vi "Log Data.vi"(8 "error in (no error)":errorcluster, 9 "DataQueues":refnum<queue>[](array[refnum]), 10 "UI":refnum<queue>, 11 "Config":T1={"Hardware Configuration"={"Camera Configuration"={"Setting"={"Expouse"=0.0, "Frames"=0.0, "Interval"=0.0, "ROI"={"x"=0.0, "y"=0.0, "width"=0.0, "height"=0.0}, "Binning"={"Binning X"=0.0, "Binning Y"=0.0}}, "Resource"={"CameraRef"=refnum, "LibraryRef"=refnum, "ImagesArray"=[]}}, "Stages Configuration"={"Resource"={"NanoStage Ref"=0, "MicroStage Ref"=0, "TirfLock Ref"=0}, "SettingValues"={"NanoState"={"Time"=0.0, "X"=0.0, "Y"=0.0, "Z"=0.0}, "MicroState"={"Time 2"=0.0, "Z"=0.0, "IsEPISet?"=FALSE}, "TirfLock"={"Time"=0.0, "X"=0.0, "Y"=0.0, "Sum"=0.0, "Calbrate"=0.0, "LockedTarget"=0.0, "Kp"=0.0, "Ki"=0.0, "Avg"=0.0}}}, "Lasers Configuration"={"SettingValues"={"405 Power"=0.0, "488 Power"=0.0, "532 Power"=0.0, "561 Power"=0.0, "647 Power"=0.0, "785 Power"=0.0}, "Resource"={"Library Ref"=refnum, "Lasers Ref"={"405 Ref"=refnum, "488 Ref"=refnum, "532 Ref"=refnum, "561 Ref"=refnum, "647 Ref"=refnum, "785 Ref"=refnum}}}}, "Logging Configuration"={"Log File Base Folder"=path "", "FileSurfix"="", "TiffFileFullPath"=path "", "TimeStampFile Ref"=refnum, "NoteFileRef"=refnum, "QuickNoteInfo"=""}, "HardWare Status"={"CameraAndStages"={"Camera"=FALSE, "NanoStage"=FALSE, "MicroStage"=FALSE, "TIRFLock"=FALSE}, "Lasers"={"IsConnected"={"405"=FALSE, "488"=FALSE, "532"=FALSE, "561"=FALSE, "647"=FALSE, "785"=FALSE}, "IsOpened"={"405"=FALSE, "488"=FALSE, "532"=FALSE, "561"=FALSE, "647"=FALSE, "785"=FALSE}}}, "CallBack Ref"={"LiveAcq callback Ref"=refnum, "AlbumAcq callback Ref"=refnum, "SequenceAcq callback Ref"=refnum, "Camera Status callback Ref"=refnum}, "Acqusition Control"={"Images Saving"={"StreamToDisk?"=FALSE, "SingleStack?"=FALSE, "Alert when finish?"=FALSE}, "Debug"={"Global Debug"=FALSE, "Global Debug Value"=0.0}}, "Runtime Parameters"={"Scale Bar"=TRUE, "ScaleBarSize"=10.0, "XYIncreatement+"=40.0, "ZIncreatement++"=5.0, "Autostretch"=FALSE, "ZIncreatement+"=0.2, "MicroStage+"=100.0, "XYIncreatement++"=80.0}} {"Runtime Parameters"."XYIncreatement++" format="%#_13g"; "Runtime Parameters"."MicroStage+" format="%#_13g"; "Runtime Parameters"."ZIncreatement+" format="%#_13g"; "Runtime Parameters"."ZIncreatement++" format="%#_13g"; "Runtime Parameters"."XYIncreatement+" format="%#_13g"; "Runtime Parameters"."ScaleBarSize" format="%#_13g"; "Hardware Configuration"."Lasers Configuration"."SettingValues"."785 Power" format="%.1f"; "Hardware Configuration"."Lasers Configuration"."SettingValues"."647 Power" format="%.1f"; "Hardware Configuration"."Lasers Configuration"."SettingValues"."561 Power" format="%.1f"}) -> (0 "error out":errorcluster)   [LabVIEW 2020, in "Logging.lvlib"]
doc: "This VI uses the TDMS Write function to write data to a TDMS file."
uses:
  Logging.lvlib
  Settings/System Running Settings.ctl
  HardwareAdapter/Support/Hardware Configuration.ctl
  HardwareAdapter/Support/Camera Configuration.ctl
  controls/ROI.ctl
  D:/Daguan/Development/RM21-MMicrosopeSource/HardwareAdapter/Camera/Dependencies/PVCamNET.dll
  HardwareAdapter/Camera/Dependencies/PVCamNET.dll
  <vilib>/vision/Image Controls.llb/IMAQ Image.ctl
  D:/Daguan/Development/RM21-MMicrosopeSource/HardwareAdapter/Lasers/Dependencies/Oxxius_Boxx.dll
  HardwareAdapter/Lasers/Dependencies/Oxxius_Boxx.dll
  Logging Configuration.ctl
  controls/DeviceStatusCtl.ctl
  controls/CallBack Refs.ctl
  Acquisition/Acquisition Control.ctl
  controls/Runtime Parameters.ctl
  support/Message Queue/Message Cluster.ctl
  controls/Image MatadataCtl.ctl
  Global.vi
  Settings/Settings.lvlib
  support/Message Queue/Message Queue.lvlib
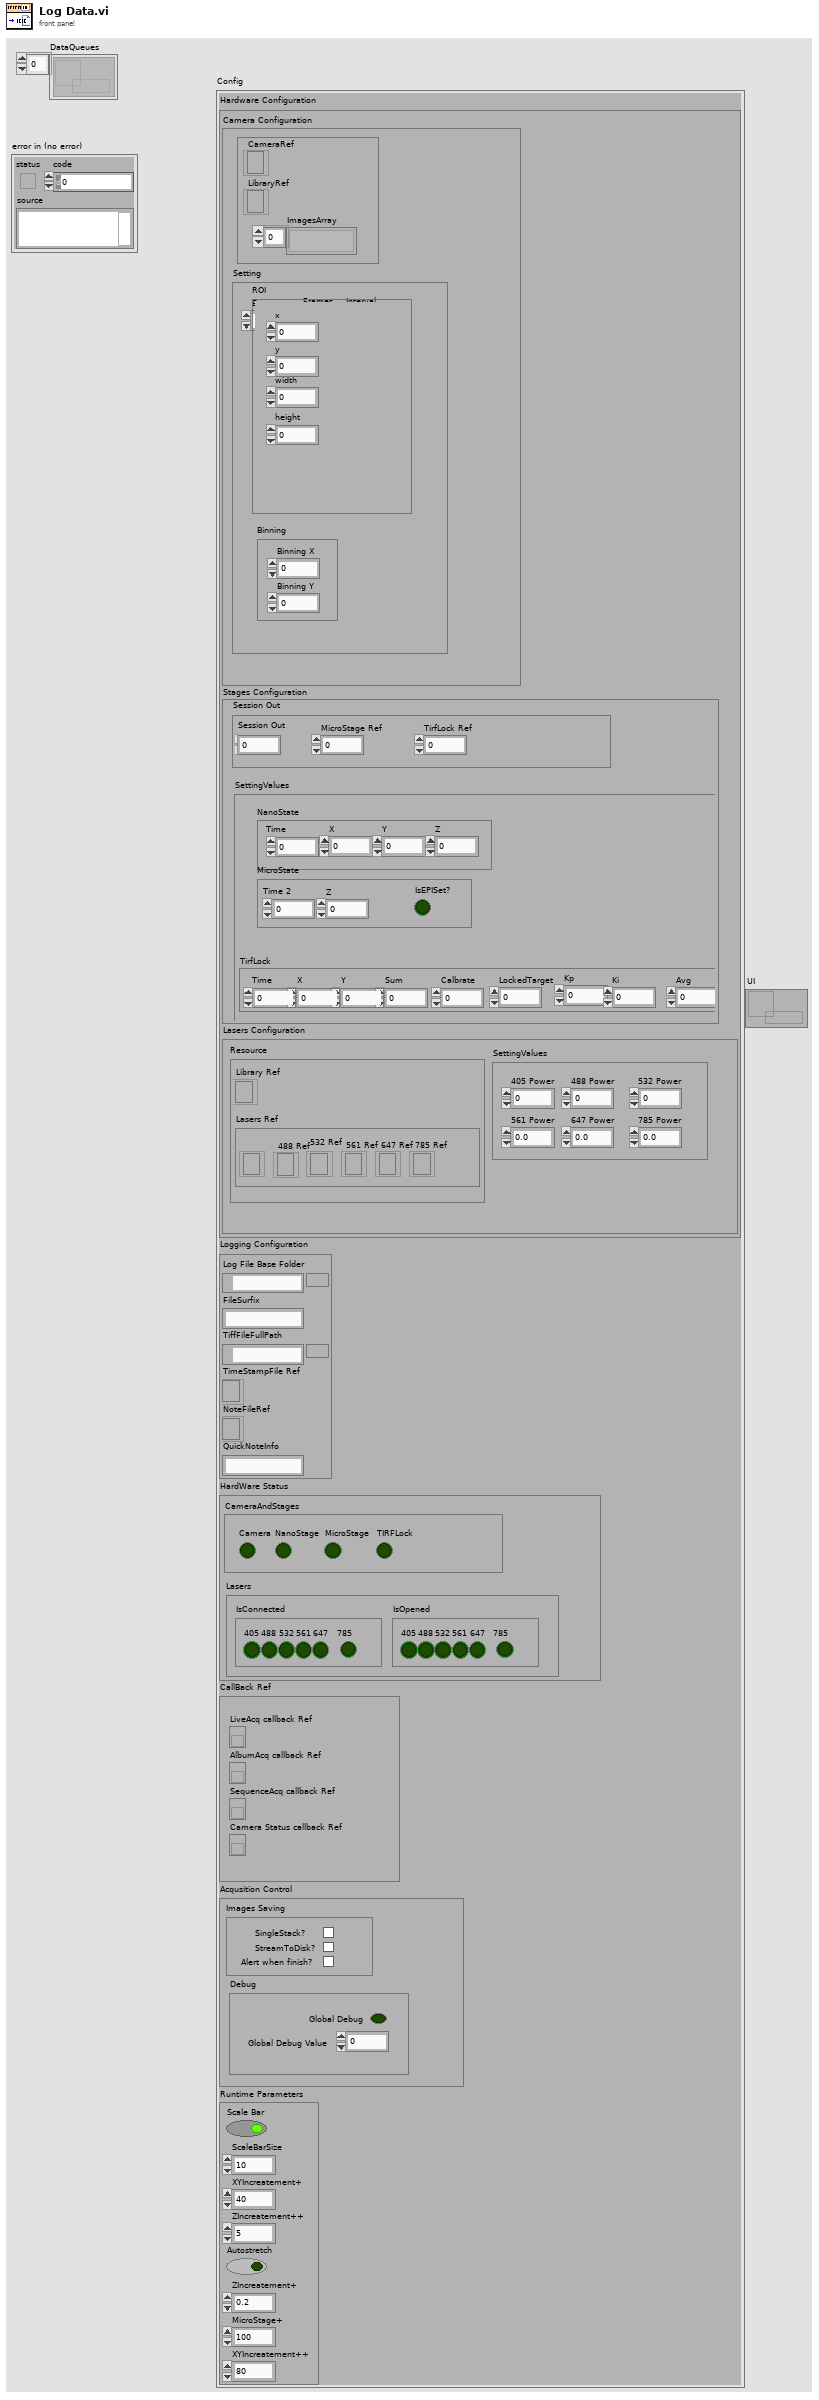
[diagram p1: front panel]
types:
  T1 = typedef "Settings.lvlib/System Running Settings.ctl" = cluster{"Hardware Configuration":T2, "Logging Configuration":T6, "HardWare Status":cluster{"CameraAndStages":T7, "Lasers":cluster{"IsConnected":cluster{"405":bool, "488":bool, "532":bool, "561":bool, "647":bool, "785":bool}, "IsOpened":cluster{"405":bool, "488":bool, "532":bool, "561":bool, "647":bool, "785":bool}}}, "CallBack Ref":T8, "Acqusition Control":T9, "Runtime Parameters":T10}
  T2 = typedef "Hardware Configuration.ctl" = cluster{"Camera Configuration":T3, "Stages Configuration":cluster{"Resource":cluster{"NanoStage Ref":i32, "MicroStage Ref":i32, "TirfLock Ref":i32}, "SettingValues":cluster{"NanoState":cluster{"Time":dbl, "X":dbl, "Y":dbl, "Z":dbl}, "MicroState":cluster{"Time 2":dbl, "Z":dbl, "IsEPISet?":bool}, "TirfLock":cluster{"Time":dbl, "X":dbl, "Y":dbl, "Sum":dbl, "Calbrate":dbl, "LockedTarget":dbl, "Kp":dbl, "Ki":dbl, "Avg":dbl}}}, "Lasers Configuration":cluster{"SettingValues":cluster{"405 Power":sgl, "488 Power":sgl, "532 Power":sgl, "561 Power":sgl, "647 Power":sgl, "785 Power":sgl}, "Resource":cluster{"Library Ref":refnum<k24>, "Lasers Ref":cluster{"405 Ref":refnum<k24>, "488 Ref":refnum<k24>, "532 Ref":refnum<k24>, "561 Ref":refnum<k24>, "647 Ref":refnum<k24>, "785 Ref":refnum<k24>}}}}
  T3 = typedef "Camera Configuration.ctl" = cluster{"Setting":cluster{"Expouse":dbl, "Frames":dbl, "Interval":dbl, "ROI":T4, "Binning":cluster{"Binning X":dbl, "Binning Y":dbl}}, "Resource":cluster{"CameraRef":refnum<k24>, "LibraryRef":refnum<k24>, "ImagesArray":T5[]}}
  T4 = typedef "ROI.ctl" = cluster{"x":dbl, "y":dbl, "width":dbl, "height":dbl}
  T5 = typedef "IMAQ Image.ctl" = refnum<image>
  T6 = typedef "Logging.lvlib/Logging Configuration.ctl" = cluster{"Log File Base Folder":path, "FileSurfix":string, "TiffFileFullPath":path, "TimeStampFile Ref":refnum<file>, "NoteFileRef":refnum<file>, "QuickNoteInfo":string}
  T7 = typedef "DeviceStatusCtl.ctl" = cluster{"Camera":bool, "NanoStage":bool, "MicroStage":bool, "TIRFLock":bool}
  T8 = typedef "CallBack Refs.ctl" = cluster{"LiveAcq callback Ref":refnum<k27>, "AlbumAcq callback Ref":refnum<k27>, "SequenceAcq callback Ref":refnum<k27>, "Camera Status callback Ref":refnum<k27>}
  T9 = typedef "Acquisition Control.ctl" = cluster{"Images Saving":cluster{"StreamToDisk?":bool, "SingleStack?":bool, "Alert when finish?":bool}, "Debug":cluster{"Global Debug":bool, "Global Debug Value":dbl}}
  T10 = typedef "Runtime Parameters.ctl" = cluster{"Scale Bar":bool, "ScaleBarSize":dbl, "XYIncreatement+":dbl, "ZIncreatement++":dbl, "Autostretch":bool, "ZIncreatement+":dbl, "MicroStage+":dbl, "XYIncreatement++":dbl}
  T11 = typedef "Image MatadataCtl.ctl" = cluster{"EofTimeStamp(Acq)":dbl, "Image":T5, "Histogram":u32[], "MeanValue":dbl, "Min":u32, "Max":u32, "EofTimeStamp(Album)":dbl, "Fps":dbl, "BufferIndex":u32, "DroppedFrames":u32, "SaveImage?":bool}
  T12 = cluster{"DataQueues[0]":refnum<queue>, "DataQueues[1]":refnum<queue>, "DataQueues[2]":refnum<queue>, "DataQueues[3]":refnum<queue>, "DataQueues[4]":refnum<queue>, "DataQueues[5]":refnum<queue>, "DataQueues[6]":refnum<queue>, "DataQueues[7]":refnum<queue>, "DataQueues[8]":refnum<queue>}
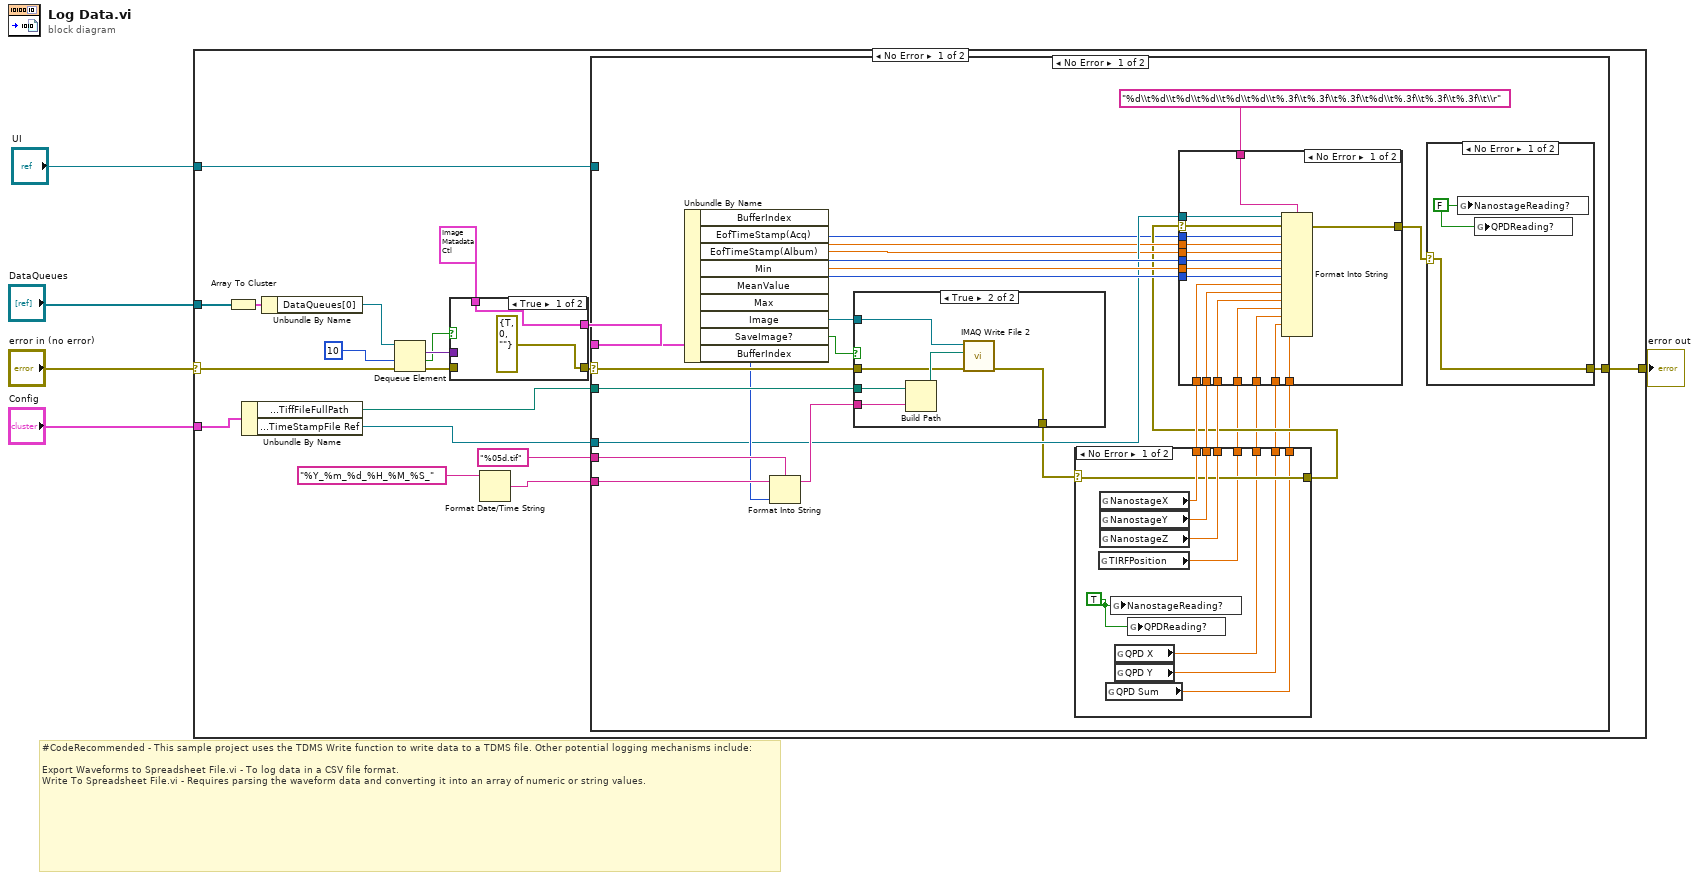
[diagram p0: block diagram]
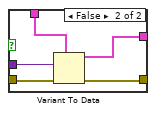
[diagram p2: hidden frame]
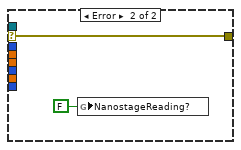
[diagram p5: hidden frame]
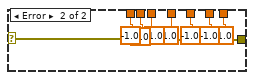
[diagram p6: hidden frame]
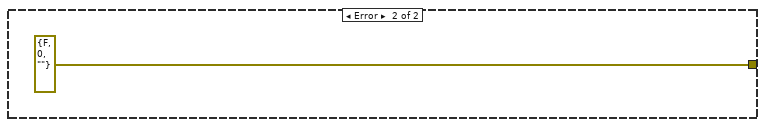
[diagram p7: hidden frame]
diagram:
  # "#CodeRecommended - This sample project uses the TDMS Write function to write data to a TDMS file. Other potential logging mechanisms include:\n\nExport Waveforms to Spreadsheet File.vi - To log data in a CSV file format.\nWrite To Spreadsheet File.vi - Requires parsing the waveform data and converting it into an array of numeric or string values."
  n1 = case shown="No Error" "error in (no error)" {
    selector: "error in (no error)" -> [w24 w107]
    tunnel: "Config" -> [w6 _]
    tunnel: "DataQueues" -> [w23 _]
    tunnel: [w19 w107] -> w5
    tunnel: "UI" -> [w7 _]
    frame No Error {
      n2 = Array To Cluster(array=w23) -> (cluster=w22:T12)
      n3 = Unbundle By Name(w6) -> ("Logging Configuration.TiffFileFullPath"=w16:path, "Logging Configuration.TimeStampFile Ref"=w8:refnum<file>)
      n4 = Unbundle By Name(w22) -> ("DataQueues[0]"=w12:refnum<queue>)
      n5 = Dequeue Element(queue=w12, timeout in ms (-1)=10, error in (no error)=w24) -> (element=w21:variant, timed out?=w9:bool, error out=w20:errorcluster)  [unwired: 1 out]
      n6 = case shown="True" w9 {
        tunnel: w21 -> [_ w31]
        tunnel: w20 -> [_ w30]
        tunnel: [w26 w29] -> w18
        tunnel: T11 {"EofTimeStamp(Acq)"=0.0, "Image"=refnum, "Histogram"=[], "MeanValue"=0.0, "Min"=0, "Max"=0, "EofTimeStamp(Album)"=0.0, "Fps"=0.0, "BufferIndex"=0, "DroppedFrames"=0, "SaveImage?"=FALSE} ("RawImage") -> [w26 w28]
        tunnel: [errorcluster {"status"=TRUE, "code"=0, "source"=""} ("error out") w27] -> w11
        frame True {
        }
        frame False {
          n7 = Variant To Data(error in=w30, type=w28, Variant=w31) -> (data=w29:T11, error out=w27:errorcluster)
        }
      }
      n8 = Format Date/Time String(time format string (%c)="%Y_%m_%d_%H_%M_%S_") -> (date/time string=w15:string)  [unwired: 2 in]
      n9 = case shown="No Error" w11 {
        selector: w11 -> [w53 _]
        tunnel: [w34 errorcluster {"status"=FALSE, "code"=0, "source"=""} ("error out")] -> w19
        tunnel: w18 -> [w59 _]
        tunnel: w16 -> [w58 _]
        tunnel: w15 -> [w57 _]
        tunnel: "%05d.tif" ("format string") -> [w56 _]
        tunnel: w8 -> [w47 _]
        tunnel: w7 -> [_ _]
        frame No Error {
          n10 = Unbundle By Name(w59) -> ("BufferIndex"=w33:u32, "EofTimeStamp(Acq)"=w46:dbl, "EofTimeStamp(Album)"=w45:dbl, "Min"=w52:u32, "MeanValue"=w51:dbl, "Max"=w50:u32, "Image"=w49:T5, "SaveImage?"=w36:bool, "BufferIndex"=w48:u32)
          n11 = Format Into String(format string=w56, initial string=w57, w48) -> (resulting string=w55:string)  [unwired: 1 in, 1 out]
          n12 = case shown="True" w36 {
            tunnel: w58 -> [_ w69]
            tunnel: w55 -> [_ w67]
            tunnel: w53 -> [w63 w66]
            tunnel: w49 -> [_ w65]
            tunnel: [w63 w64] -> w41
            frame False {
            }
            frame True {
              n13 = Build Path(base path=w69, name or relative path=w67) -> (appended path=w68:path)
              n14 = call-poly "IMAQ Write File 2"("error in (no error)"=w66, "File Path"=w68, "Image"=w65) -> ("error out"=w64:errorcluster)  [unwired: 7 in, 1 out]
            }
          }
          n15 = case shown="No Error" w41 {
            selector: w41 -> [w94 w105]
            tunnel: [w97 -1.0 ("NanostageX")] -> w44
            tunnel: [w96 -1.0 ("NanostageY")] -> w43
            tunnel: [w95 -1.0 ("NanostageZ")] -> w42
            tunnel: [w94 w105] -> w40
            tunnel: [w93 -1.0 ("NanostageX")] -> w39
            tunnel: [w92 -1.0 ("NanostageY")] -> w38
            tunnel: [w91 -1.0 ("NanostageZ")] -> w37
            tunnel: [w89 -1.0 ("TIRFPosition")] -> w32
            frame No Error {
              w90 = TRUE ("NanostageReading?")
              n16 = global read "Global.vi" "TIRFPosition"() -> (w89:dbl)
              n17 = global read "Global.vi" "NanostageX"() -> (w97:dbl)
              n18 = global read "Global.vi" "NanostageY"() -> (w96:dbl)
              n19 = global read "Global.vi" "NanostageZ"() -> (w95:dbl)
              n20 = global read "Global.vi" "QPD Sum"() -> (w91:dbl)
              n21 = global write "Global.vi" "NanostageReading?"(w90) -> ()
              n22 = global read "Global.vi" "QPD X"() -> (w93:dbl)
              n23 = global read "Global.vi" "QPD Y"() -> (w92:dbl)
              n24 = global write "Global.vi" "QPDReading?"(w90) -> ()
            }
            frame Error {
            }
          }
          n25 = case shown="No Error" w40 {
            selector: w40 -> [w74 w88]
            tunnel: "%d\\t%d\\t%d\\t%d\\t%d\\t%d\\t%.3f\\t%.3f\\t%.3f\\t%d\\t%.3f\\t%.3f\\t%.3f\\t\\r" ("format string") -> [w86 _]
            tunnel: [w85 w88] -> w35
            tunnel: w33 -> [w84 _]
            tunnel: w52 -> [w83 _]
            tunnel: w51 -> [w82 _]
            tunnel: w50 -> [w81 _]
            tunnel: w47 -> [w80 _]
            tunnel: w46 -> [w79 _]
            tunnel: w45 -> [w78 _]
            tunnel: w44 -> [w77 _]
            tunnel: w43 -> [w76 _]
            tunnel: w42 -> [w75 _]
            tunnel: w39 -> [w73 _]
            tunnel: w38 -> [w72 _]
            tunnel: w37 -> [w71 _]
            tunnel: w32 -> [w70 _]
            frame No Error {
              n26 = Format Into String(format string=w86, initial string=w80, error in=w74, w84, w79, w78, w83, w82, w81, w77, w76, w75, w70, w73, w72, w71) -> (error out=w85:errorcluster)  [unwired: 1 out]
            }
            frame Error {
              n27 = global write "Global.vi" "NanostageReading?"(FALSE ("NanostageReading?")) -> ()
            }
          }
          n28 = case shown="No Error" w35 {
            selector: w35 -> [w61 w62]
            tunnel: [w61 w62] -> w34
            frame No Error {
              w60 = FALSE ("NanostageReading?")
              n29 = global write "Global.vi" "NanostageReading?"(w60) -> ()
              n30 = global write "Global.vi" "QPDReading?"(w60) -> ()
            }
            frame Error {
            }
          }
        }
        frame Error {
        }
      }
    }
    frame Error {
    }
  }
  "error out" <- w5
